vi "Colour.vi"(9 "result":string, 11 "colourRef":refnum<vi>) -> (3 "colourRef 2":refnum<vi>)   [LabVIEW 2013]
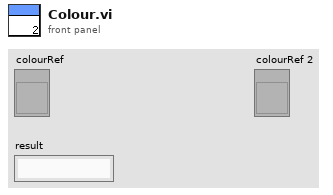
[diagram p1: front panel]
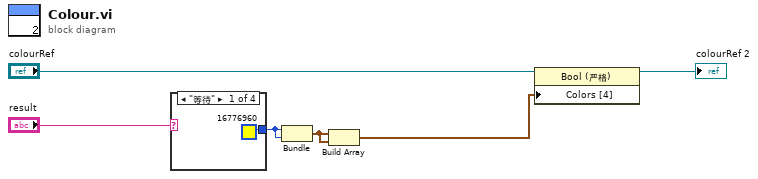
[diagram p0: block diagram]
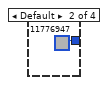
[diagram p2: hidden frame]
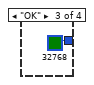
[diagram p3: hidden frame]
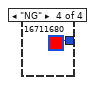
[diagram p4: hidden frame]
diagram:
  n1 = case shown="\"等待\"" "result" {
    tunnel: [u32 16776960 u32 11776947 u32 32768 u32 16711680] -> w6
    frame "等待" {
    }
    frame Default {
    }
    frame "OK" {
    }
    frame "NG" {
    }
  }
  n2 = Bundle(w6, w6) -> (w3:cluster{u32, u32})  [unwired: 1 in]
  n3 = Build Array(w3, w3) -> (w5:cluster{u32, u32}[])
  n4 = property on="属性节点" class="Bool (严格)"(reference="colourRef", "Colors [4]"=w5) -> (reference out=→"colourRef 2":refnum<vi>)  [unwired: 1 in, 1 out]
